vi "constants.vi"() -> (2 "?":T1)   [LabVIEW 2015]
doc: "This VI outputs a cluster of clusters that have constants for the intialization process. Use the Unbundle by name to access the constants."
uses:
  constants.ctl
  <vilib>/Rock Robotics/SystemInterfaces/DIO/FPGA_DIOPWMChannel.ctl
panel:
  # "ShooterMotors"
  # "DriveMotors- CAN Bus"
  # "PWM"
  # "ClimberMotors"
  # "CAN Bus"
  # "CAN Bus"
  # "PWM"
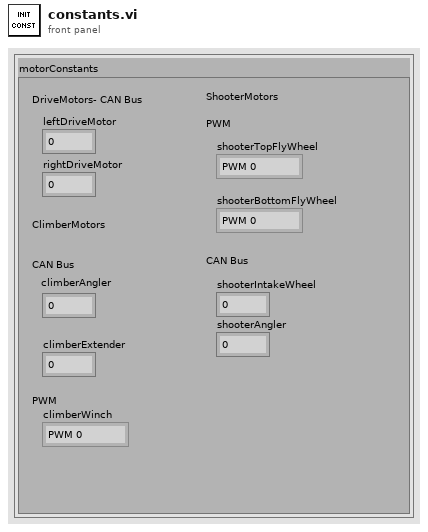
[diagram p1: front panel]
types:
  T1 = typedef "constants.ctl" = cluster{"motorConstants":cluster{"leftDriveMotor":i32, "rightDriveMotor":i32, "climberAngler":i32, "climberWinch":T2, "shooterTopFlyWheel":T2, "shooterBottomFlyWheel":T2, "climberExtender":i32, "shooterIntakeWheel":i32, "shooterAngler":i32}}
  T2 = typedef "FPGA_DIOPWMChannel.ctl" = enum8{"PWM 0", "PWM 1", "PWM 2", "PWM 3", "PWM 4", "PWM 5", "PWM 6", "PWM 7", "PWM 8", "PWM 9", "PWM MXP 0", "PWM MXP 1", "PWM MXP 2", "PWM MXP 3", "PWM MXP 4", "PWM MXP 5", "PWM MXP 6", "PWM MXP 7", "PWM MXP 8", "PWM MXP 9", "Invalid"}
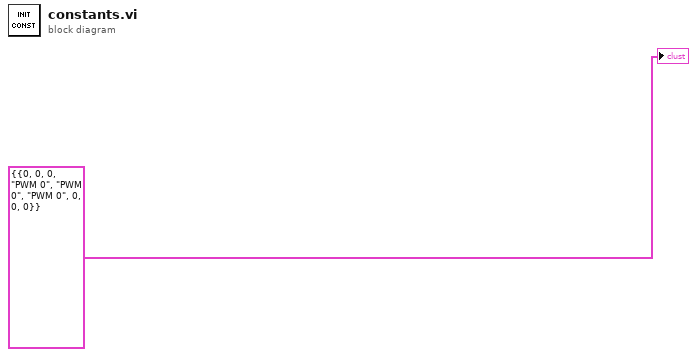
[diagram p0: block diagram]
diagram:
  "?" <- T1 {"motorConstants"={"leftDriveMotor"=0, "rightDriveMotor"=0, "climberAngler"=0, "climberWinch"=enum."PWM 0", "shooterTopFlyWheel"=enum."PWM 0", "shooterBottomFlyWheel"=enum."PWM 0", "climberExtender"=0, "shooterIntakeWheel"=0, "shooterAngler"=0}}
